vi "Stop Periodic Replies Checks.vi"(8 "error in (no error)":errorcluster, 11 "Tamer in":refnum<class "Tamer.lvclass">) -> (0 "error out":errorcluster, 3 "Tamer out":refnum<class "Tamer.lvclass">)   [LabVIEW 2020, in "Tamer.lvlib" / "Tamer.lvclass"]
uses:
  Tamer.lvclass
  Ancestor/Ancestor/Infinite Message Selector.ctl
  Tamer Consumer Case Selector.ctl
  Ancestor/Ancestor/Ancestor.lvclass
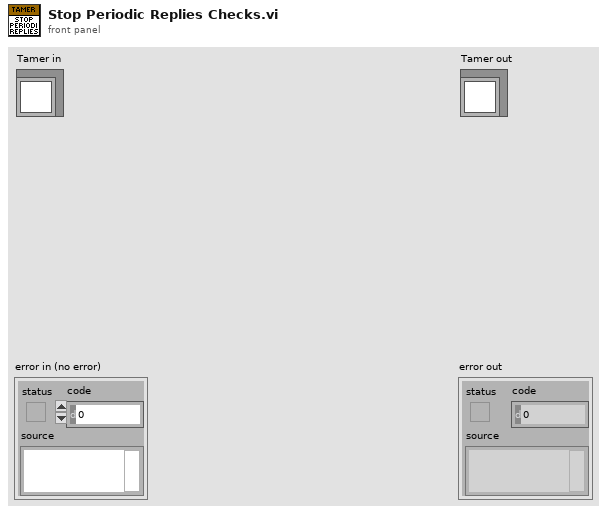
[diagram p1: front panel]
types:
  T1 = typedef "Tamer.lvlib/Tamer.lvclass/Tamer Consumer Case Selector.ctl" = enum16{"New schedule", "Initiate RUN", "Parse Schedules", "Script Checker", "Banana after Quality Check", "Update Crit Lvl", "Propagate Banana", "Reply from Guardian", "Reply from uService", "Timeout of RUN", "uService Replies Check", "Update from Monkey", "Monkey Died", "Reschedule", "Rerun", "Stop DAQ", "Stop Schedule", "Skip Run", "Kill Process", "Update GV"}
  T2 = typedef "TALOS.lvlib/Ancestor.lvlib/Ancestor.lvclass/Infinite Message Selector.ctl" = enum16{"Start", "Stop", "Check", "Flush (Stop all)", "Init"}
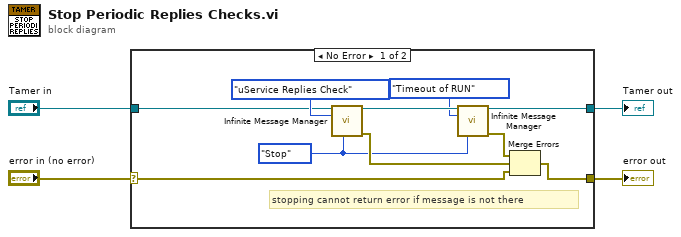
[diagram p0: block diagram]
diagram:
  n1 = case shown="No Error" "error in (no error)" {
    selector: "error in (no error)" -> [w6 w16]
    tunnel: [w5 w16] -> w3
    tunnel: [w8 w15] -> w1
    tunnel: "Tamer in" -> [w9 w15]
    frame No Error {
      w12 = Infinite_Message_Selector."Stop" ("Infinite Message Selector")
      # "stopping cannot return error if message is not there"
      n2 = call-dynamic "Infinite Message Manager.vi"("Father of all uServices in"=w9, "Consumer Case Selector"=Tamer_Consumer_Case_Selector."uService Replies Check" ("Monkey Consumer Case Selector"), "Infinite Message Selector"=w12) -> ("Father of all uServices out"=w13:refnum<class "Tamer.lvclass">, "error out"=w14:errorcluster)  [unwired: 10 in, 1 out]
      n3 = call-dynamic "Infinite Message Manager.vi"("Father of all uServices in"=w13, "Consumer Case Selector"=Tamer_Consumer_Case_Selector."Timeout of RUN" ("Monkey Consumer Case Selector"), "Infinite Message Selector"=w12) -> ("Father of all uServices out"=w8:refnum<class "Tamer.lvclass">, "error out"=w7:errorcluster)  [unwired: 10 in, 1 out]
      n4 = Merge Errors(w7, w14, w6) -> (w5:errorcluster)
    }
    frame Error {
    }
  }
  "error out" <- w3
  "Tamer out" <- w1
